vi "Dispatch Message.vi"(8 "error in (no error)":errorcluster, 10 "Server Message":refnum<class "Server Message.lvclass">, 11 "OBS in":refnum<class "OBS.lvclass">) -> (0 "error out":errorcluster, 3 "OBS out":refnum<class "OBS.lvclass">)   [LabVIEW 2022 SP3, in "obs-websocket-lv.lvlib" / "OBS.lvclass"]
uses:
  OBS.lvclass
  Server Message/Server Message.lvclass
  Hello/Hello.lvclass
  Client Message.ctl
  Client Message/Client Message.lvclass
  Response/Response.lvclass
  OBS.lvclass/OBS.ctl
  Identified/Identified.lvclass
  Identify/Identify.lvclass
  C:/dev/illuminatedg/obs-websocket-lv/obs-websocket-lv/Client Message/Client Message.lvclass
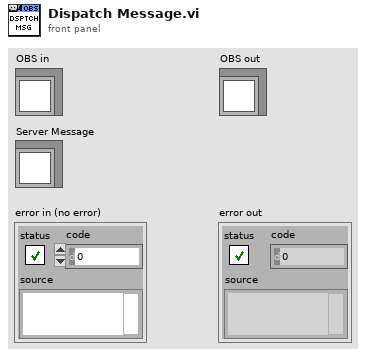
[diagram p1: front panel]
types:
  T1 = typedef "obs-websocket-lv.lvlib/Server Operation.ctl" = enum16{"Hello", "Identified", "Event", "RequestResponse", "RequestBatchResponse"}
  T2 = typedef "obs-websocket-lv.lvlib/OBS.lvclass/Client Message.ctl" = cluster{"Message":refnum<class "Client Message.lvclass">, "Response Notifier":refnum<notifier>}
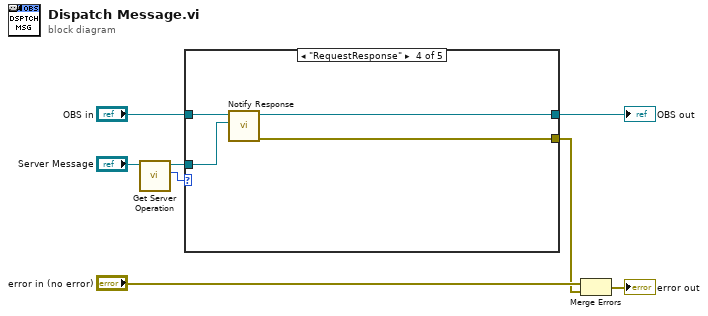
[diagram p0: block diagram]
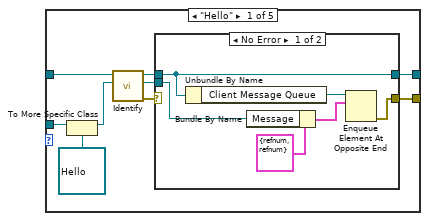
[diagram p2: hidden frame]
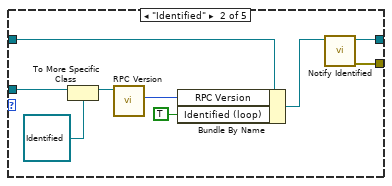
[diagram p4: hidden frame]
diagram:
  n1 = call "Get Server Operation.vi"("Server Message in"="Server Message") -> ("Server Operation"=w6:T1, "Server Message out"=w5:refnum<class "Server Message.lvclass">)  [unwired: 8 in, 1 out]
  n2 = case shown="\"RequestResponse\"" w6 {
    tunnel: w5 -> [w16 w33 _ w38 _]
    tunnel: "OBS in" -> [w17 w34 w35 w39 w40]
    tunnel: [w10 w27 w35 w37 w40] -> w3
    tunnel: [w9 w26 _ w36 _] -> w1
    frame "Hello" {
      n3 = To More Specific Class(target class=refnum<class "Hello.lvclass"> refnum ("obs-websocket-lv.lvlib:Hello.lvclass"), reference=w16) -> (specific class reference=w15:refnum<class "Hello.lvclass">)  [unwired: 1 in, 1 out]
      n4 = call "Identify.vi"("Hello Msg"=w15, "OBS in"=w17) -> ("error out"=w13:errorcluster, "Identify Msg"=w12:refnum<class "Identify.lvclass">, "OBS out"=w11:refnum<class "OBS.lvclass">)  [unwired: 7 in]
      n5 = case shown="No Error" w13 {
        selector: w13 -> [_ w25]
        tunnel: w12 -> [w18 _]
        tunnel: w11 -> [w19 w24]
        tunnel: [w19 w24] -> w10
        tunnel: [w22 w25] -> w9
        frame No Error {
          n6 = Unbundle By Name(w19) -> ("Client Message Queue"=w23:refnum<queue>)
          n7 = Bundle By Name(cluster=T2 {"Message"=refnum, "Response Notifier"=refnum} ("Client Message"), "Message"=w18) -> (w20:T2)
          n8 = Enqueue Element At Opposite End(queue=w23, element=w20) -> (error out=w22:errorcluster)  [unwired: 2 in, 2 out]
        }
        frame Error {
        }
      }
    }
    frame "Identified" {
      n9 = To More Specific Class(target class=refnum<class "Identified.lvclass"> refnum ("obs-websocket-lv.lvlib:Identified.lvclass"), reference=w33) -> (specific class reference=w31:refnum<class "Identified.lvclass">)  [unwired: 1 in, 1 out]
      n10 = call "RPC Version.vi"("Identified in"=w31) -> ("RPC Version"=w30:i32)  [unwired: 8 in, 2 out]
      n11 = Bundle By Name(cluster=w34, "RPC Version"=w30, "Identified (loop)"=TRUE) -> (w28:refnum<class "OBS.lvclass">)
      n12 = call "Notify Identified.vi"("OBS in"=w28) -> ("error out"=w26:errorcluster, "OBS out"=w27:refnum<class "OBS.lvclass">)  [unwired: 9 in]
    }
    frame "Event" {
    }
    frame "RequestResponse" {
      n13 = call "Notify Response.vi"("Server Message"=w38, "OBS in"=w39) -> ("error out"=w36:errorcluster, "OBS out"=w37:refnum<class "OBS.lvclass">)  [unwired: 8 in]
    }
    frame "RequestBatchResponse" {
    }
  }
  "OBS out" <- w3
  n14 = Merge Errors("error in (no error)", w1) -> (→"error out":errorcluster)
